vi "dataUnwrapperTRSToplevel.vi"(0 "TRSdata":u32[](array[numeric]) format="%032b", 2 "nOfSteps":i32=20, 4 "nOfScans":i32=6) -> (21 "TRSdataUntouchedOut":u32[](array[numeric]), 24 "VoltArray":u32[](array[numeric]) format="%032b")   [LabVIEW 2014]
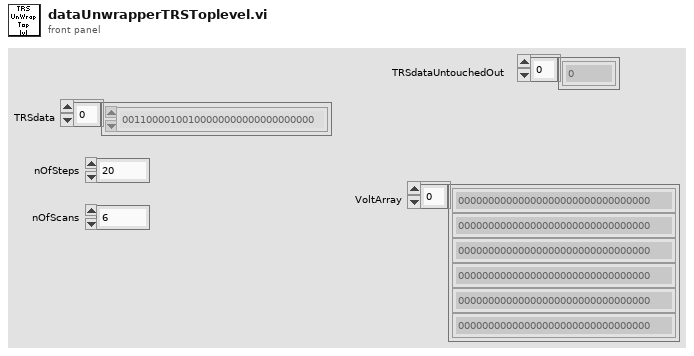
[diagram p1: front panel]
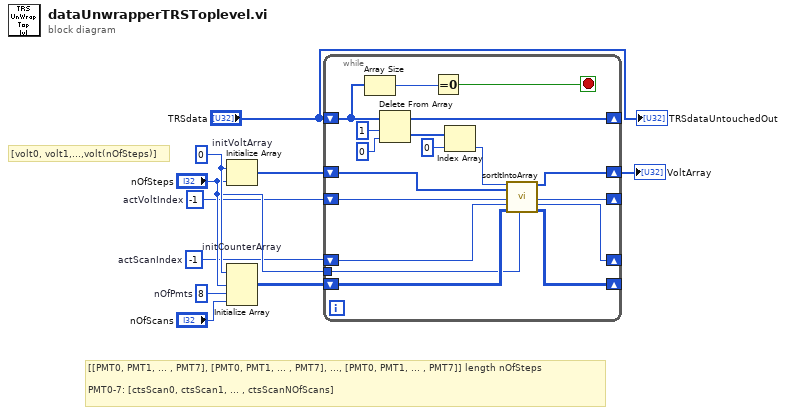
[diagram p0: block diagram]
diagram:
  w2 = -1  # actScanIndex
  w3 = -1  # actVoltIndex
  w10 = u32 0 ("element")
  w9 = 8  # nOfPmts
  # "[[PMT0, PMT1, ... , PMT7], [PMT0, PMT1, ... , PMT7], ..., [PMT0, PMT1, ... , PMT7]] length nOfSteps\n\nPMT0-7: [ctsScan0, ctsScan1, ... , ctsScanNOfScans]"
  # "[volt0, volt1,...,volt(nOfSteps)]"
  n1 = Initialize Array "initVoltArray"(w10, "nOfSteps") -> (w6:u32[])
  n2 = Initialize Array "initCounterArray"(w10, "nOfSteps", w9, "nOfScans") -> (w7:u32[][][])
  n3 = while {
    shift-right: [w26] -> _
    shift-left: "TRSdata" -> [w25]
    shift-right: [w14] -> w5
    shift-left: w6 -> [w19]
    shift-right: [w16] -> _
    shift-left: w7 -> [w17]
    shift-right: [w15] -> _
    shift-left: w3 -> [w18]
    shift-right: [w12] -> _
    shift-left: w2 -> [w13]
    tunnel: "nOfSteps" -> [w11]
    stop <- w23 stop-if-true
    n4 = Array Size(array=w25) -> (size(s)=w24:i32)
    n5 = Delete From Array(array=w25, length=1, index=0) -> (deleted portion=w22:u32[], array with subset deleted=w26:u32[])
    n6 = Equal To 0?(x=w24) -> (x = 0?=w23:bool)
    n7 = Index Array(array=w22, index=0) -> (element=w20:u32)
    n8 = call "sortItIntoArray.vi"("element"=w20, "VoltArray"=w19, "actVoltIndex"=w18, "actScanIndex"=w13, "CounterArray"=w17, "nOfSteps"=w11) -> ("VoltArrayOut"=w14:u32[], "actVoltIndexOut"=w15:i32, "actScanIndexOut"=w12:i32, "CounterArrayOut"=w16:u32[][][])  [unwired: 8 in, 2 out]
  }
  "VoltArray" <- w5
  "TRSdataUntouchedOut" <- "TRSdata"
